vi "Enable-Disable Function.vi"(8 "error in":errorcluster, 9 "Disabled":T1(ring), 10 "Labels":string[](array[string]), 11 "Map Out":map{string, refnum<vi>}(c390)) -> (0 "error out":errorcluster)   [LabVIEW 2020]
uses:
  <vilib>/Utility/error.llb/Error Cluster From Error Code.vi
  <vilib>/ErrorRing/Error Ring.xnode
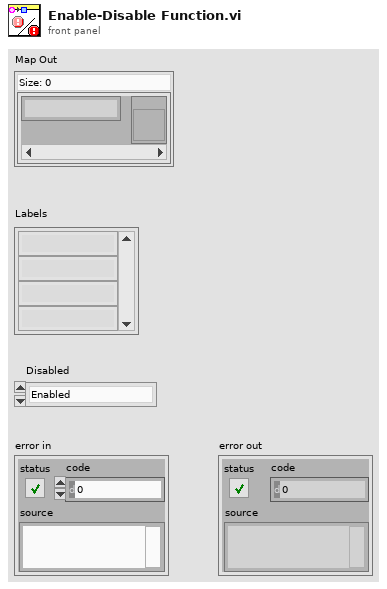
[diagram p1: front panel]
types:
  T1 = enum8{"Enabled", "Disabled", "Disabled and Grayed Out"}
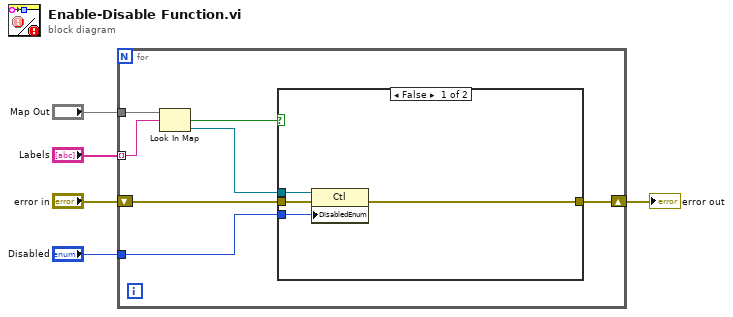
[diagram p0: block diagram]
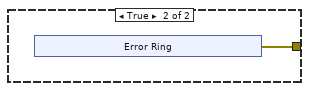
[diagram p2: hidden frame]
diagram:
  n1 = for {
    tunnel: "Labels" -> [w11] mode=indexing
    tunnel: "Map Out" -> [w12]
    shift-right: [w7] -> w2
    shift-left: "error in" -> [w8]
    tunnel: "Disabled" -> [w6]
    n2 = Look In Map(map=w12, key=w11) -> (key not found?=w9:bool, value=w10:refnum<vi>)  [unwired: 1 in]
    n3 = case shown="False" w9 {
      tunnel: w10 -> [w16 _]
      tunnel: w8 -> [w15 _]
      tunnel: [w14 w17] -> w7
      tunnel: w6 -> [w13 _]
      frame False {
        n4 = property class="Ctl"(reference=w16, error in=w15, "DisabledEnum"=w13) -> (error out=w14:errorcluster)  [unwired: 1 out]
      }
      frame True {
        n5 = xnode "Error Ring"() -> ("error out"=w17:errorcluster)
      }
    }
  }
  "error out" <- w2
